vi "Hide Subpanel.vi"(8 "error in (no error)":errorcluster, 10 "Subpanel Name":string, 11 "UI Controller in":refnum<class "UI Controller.lvclass">) -> (0 "error out":errorcluster, 3 "UI Controller out":refnum<class "UI Controller.lvclass">)   [LabVIEW 2015, in "UI Controller.lvlib" / "UI Controller.lvclass"]
uses:
  UI Controller.lvclass
  <vilib>/Utility/miscctls.llb/LVPositionTypeDef.ctl
  <vilib>/ActorFrameworkMVC/View Controller/View Controller/View Controller.lvclass
panel:
  # "NOTICE -- YOU MUST LEAVE THIS NOTICE IN PLACE.\n\nCopyright (c) 2015, LIANG LIU Shawn.Liu.cn@gmail.com\nAll rights reserved.\n\nRedistribution and use in source and binary forms, with or without modification, are permitted provided that the following conditions are met:\n-Redistributions of source code must retain the above copyright notice, this list of conditions and the following disclaimer.\n-Redistributions in binary form must reproduce the above copyright notice, this list of conditions and the following disclaimer in the documentation and/or other materials provided with the distribution.\n-Neither the name of the eLp nor the names of its contributors may be used to endorse or promote products derived from this software without specific prior written permission.\n\nTHIS SOFTWARE IS PROVIDED BY THE COPYRIGHT HOLDERS AND CONTRIBUTORS \"AS IS\" AND ANY EXPRESS OR IMPLIED WARRANTIES, INCLUDING, BUT NOT LIMITED TO, THE IMPLIED WARRANTIES OF MERCHANTABILITY AND FITNESS FOR A PARTICULAR PURPOSE ARE DISCLAIMED. IN NO EVENT SHALL THE COPYRIGHT HOLDER OR CONTRIBUTORS BE LIABLE FOR ANY DIRECT, INDIRECT, INCIDENTAL, SPECIAL, EXEMPLARY, OR CONSEQUENTIAL DAMAGES (INCLUDING, BUT NOT LIMITED TO, PROCUREMENT OF SUBSTITUTE GOODS OR SERVICES; LOSS OF USE, DATA, OR PROFITS; OR BUSINESS INTERRUPTION) HOWEVER CAUSED AND ON ANY THEORY OF LIABILITY, WHETHER IN CONTRACT, STRICT LIABILITY, OR TORT (INCLUDING NEGLIGENCE OR OTHERWISE) ARISING IN ANY WAY OUT OF THE USE OF THIS SOFTWARE, EVEN IF ADVISED OF THE POSSIBILITY OF SUCH DAMAGE."
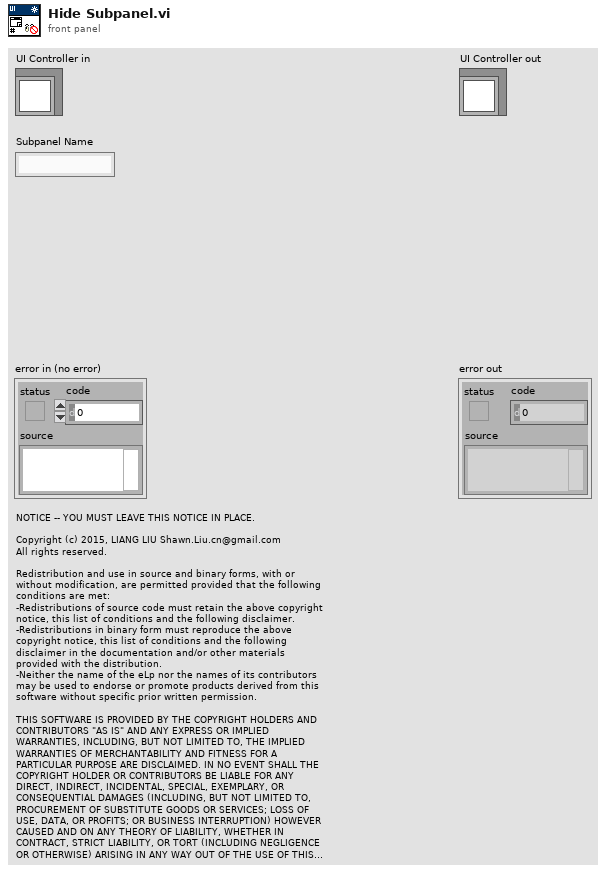
[diagram p1: front panel]
types:
  T1 = typedef "LVPositionTypeDef.ctl" = cluster{"Left":i32, "Top":i32}
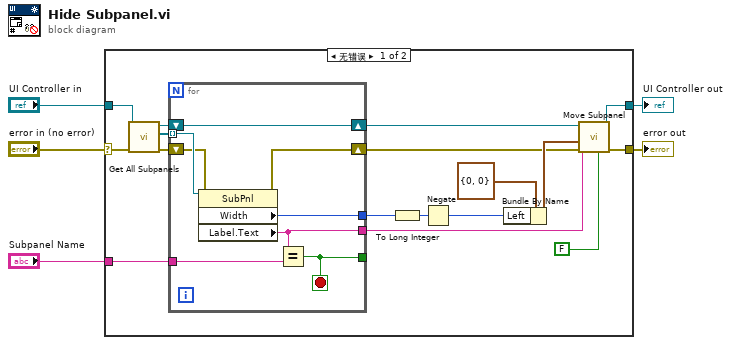
[diagram p0: block diagram]
diagram:
  n1 = case shown="无错误" "error in (no error)" {
    selector: "error in (no error)" -> [w9 w32]
    tunnel: "Subpanel Name" -> [w19 _]
    tunnel: [w8 w32] -> w3
    tunnel: [w7 w31] -> w2
    tunnel: "UI Controller in" -> [w6 w31]
    frame No Error {
      n2 = call <vilib>:"Get All Subpanels.vi"("error in (no error)"=w9, "View Controller in"=w6) -> ("error out"=w11:errorcluster, "Subpanels"=w20:refnum<vi>[], "View Controller out"=w22:refnum<class "UI Controller.lvclass">)  [unwired: 7 in]
      n3 = for {
        shift-right: [w30] -> w21
        shift-left: w22 -> [w30]
        tunnel: w20 -> [w29] mode=indexing
        tunnel: w19 -> [w28]
        tunnel: [w27] -> w15
        tunnel: [w26] -> _
        tunnel: [w25] -> w18
        shift-right: [w23] -> w10
        shift-left: w11 -> [w24]
        stop <- w26 stop-if-true
        n4 = property class="SubPnl"(reference=w29, error in=w24) -> (error out=w23:errorcluster, "Width"=w27:u32, "Label.Text"=w25:string)  [unwired: 1 out]
        n5 = Equal?(x=w25, y=w28) -> (x = y?=w26:bool)
      }
      n6 = To Long Integer(number=w15) -> (32bit integer=w14:i32)
      n7 = Negate(x=w14) -> (-x=w13:i32)
      n8 = Bundle By Name(cluster=T1 {"Left"=0, "Top"=0} ("Position"), "Left"=w13) -> (w16:T1)
      n9 = call-dynamic "Move Subpanel.vi"("Visible (True)"=FALSE, "error in (no error)"=w10, "Position"=w16, "Subpanel Name"=w18, "UI Controller in"=w21) -> ("error out"=w8:errorcluster, "UI Controller out"=w7:refnum<class "UI Controller.lvclass">)  [unwired: 5 in]
    }
    frame Error {
    }
  }
  "error out" <- w3
  "UI Controller out" <- w2
